vi "Trampsimple.vi"(6 "stop":bool, 7 "Rate [K/min]":dbl=0.05, 8 "delta K":dbl=0.2, 9 "T stop [K]":dbl=10.0 min=0.25 max=400.0, 10 "T start [K]":dbl=4.0 min=0.25 max=400.0, 11 "ITCSignal":T1={"ITC"=0, "Signal"=enum."Sensor 3"}) -> (2 "Finished":bool, 3 "ITCSignal out":T1={"ITC"=0, "Signal"=enum."Sensor 1"})   [LabVIEW 2011]
uses:
  Kelvinox drivers/ITCAPPS - Copie.LLB/ITCSignal.ctl
  Kelvinox drivers/ITCAPPS.LLB/ITCSignals.ctl
panel:
  out "Current T":dbl
  out "sign":i32=4 min=2 max=400
  out "timer":u32
  # "Sweep T"
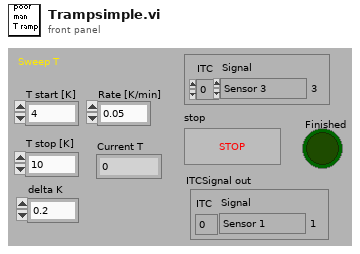
[diagram p1: front panel]
types:
  T1 = typedef "ITCSignal.ctl" = cluster{"ITC":u16, "Signal":T2}
  T2 = typedef "ITCSignals.ctl" = enum16{"Setpoint", "Sensor 1", "Sensor 2", "Sensor 3", "Needle Valve %", "Heater %"}
  T3 = typedef "ITCSetup.ctl" = cluster{"Description":string, "IO Info":T4}
  T4 = typedef "ITCIO.ctl" = cluster{"Address":T5, "Version":T6, "Ch 1 dec places":i16, "Ch 2 dec places":i16, "Ch 3 dec places":i16, "Ch1 Name":string, "Ch2 Name":string, "Ch3 Name":string}
  T5 = typedef "OxfordAddress.ctl" = cluster{"Com Port":i32, "ISOBUS Address":i32, "GPIB Address":i16, "Communication":enum16{"RS232", "ISOBUS", "GPIB", "Gateway"}}
  T6 = typedef "ITCVersion.ctl" = enum16{"ITC502", "ITC503", "ITC601"}
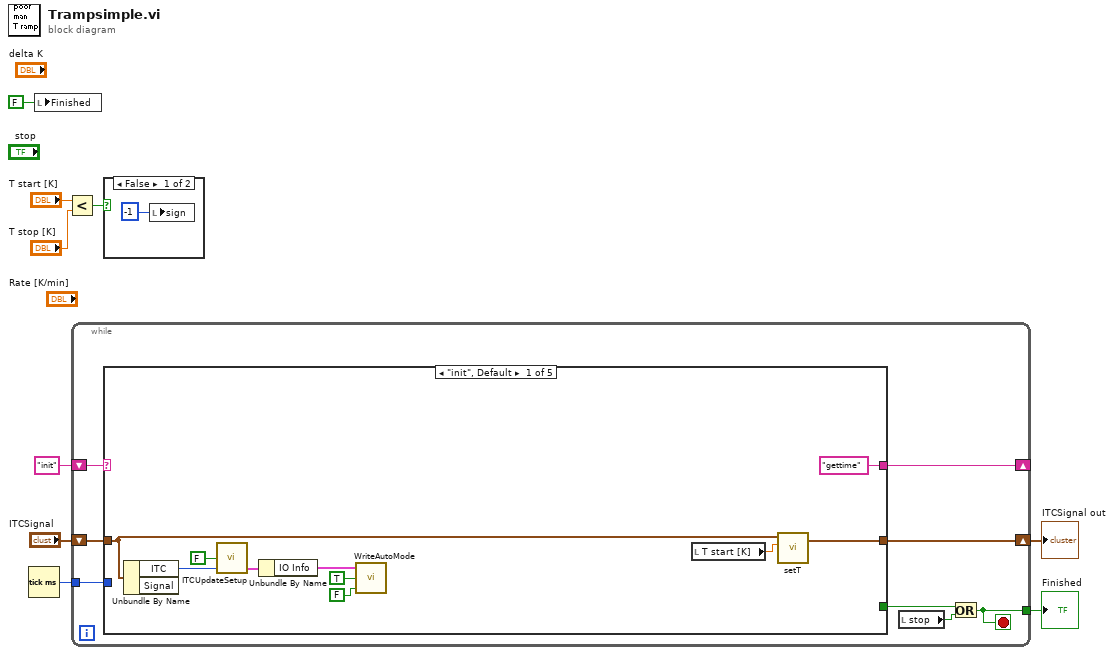
[diagram p0: block diagram]
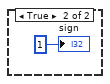
[diagram p2: hidden frame]
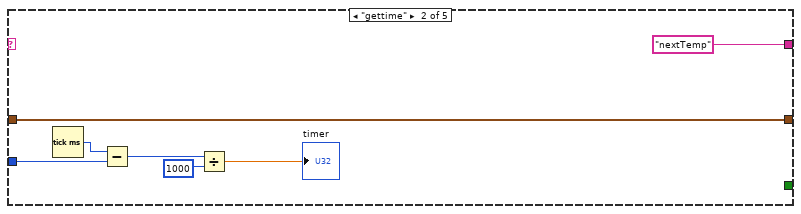
[diagram p3: hidden frame]
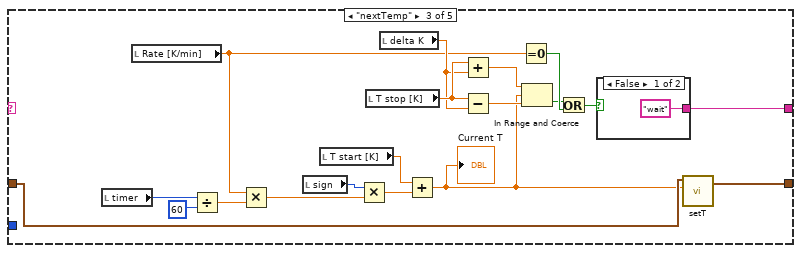
[diagram p4: hidden frame]
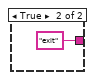
[diagram p5: hidden frame]
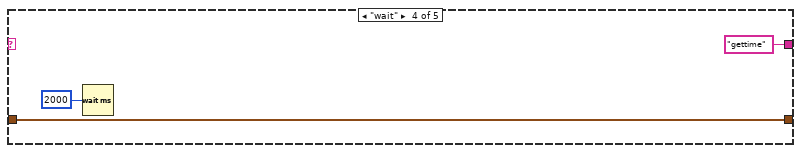
[diagram p6: hidden frame]
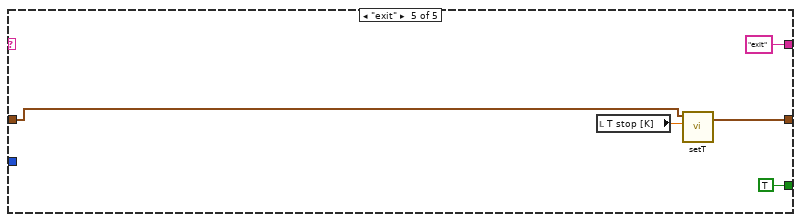
[diagram p7: hidden frame]
diagram:
  n1 = Tick Count (ms)() -> (millisecond timer value=w8:u32)
  n2 = local write "Finished"(FALSE ("Finished")) -> ()
  n3 = Less?(x="T start [K]", y="T stop [K]") -> (x < y?=w4:bool)
  n4 = while {
    shift-right: [w13] -> _
    shift-left: "init" -> [w17]
    tunnel: w8 -> [w16]
    shift-right: [w14] -> w2
    shift-left: "ITCSignal" -> [w15]
    tunnel: [w11] -> w3
    stop <- w11 stop-if-true
    n5 = case shown="\"init\", Default" w17 {
      tunnel: w16 -> [_ w33 _ _ _]
      tunnel: w15 -> [w21 w28 w49 w56 w60]
      tunnel: [w26 w28 w48 w56 w59] -> w14
      tunnel: [_ _ _ _ TRUE] -> w12
      tunnel: ["gettime" "nextTemp" w43 "gettime" "exit"] -> w13
      frame "init", Default {
        n6 = Unbundle By Name(w21) -> ("ITC"=w23:u16)  [unwired: 1 out]
        n7 = call "ITCUpdateSetup.vi"("Index"=w23, "Write to disk?"=FALSE) -> ("ITC Setup"=w22:T3)  [unwired: 2 in, 1 out]
        n8 = Unbundle By Name(w22) -> ("IO Info"=w20:T4)
        n9 = call "WriteAutoMode.vi"("Auto Needle Valve"=FALSE, "Auto Heat"=TRUE, "ITC IO Info"=w20) -> ()  [unwired: 1 out]
        n10 = local read "T start [K]"() -> (w27:dbl)
        n11 = call "setT.vi"("ITCSignal"=w21, "T target [K]"=w27) -> ("ITCSignal 2"=w26:T1)  [unwired: 3 in, 1 out]
      }
      frame "gettime" {
        n12 = Tick Count (ms)() -> (millisecond timer value=w34:u32)
        n13 = Subtract(x=w34, y=w33) -> (x-y=w32:u32)
        n14 = Divide(x=w32, y=u32 1000) -> (x/y=→"timer":dbl)
      }
      frame "nextTemp" {
        n15 = local read "timer"() -> (w41:u32)
        n16 = local read "Rate [K/min]"() -> (w38:dbl)
        n17 = Divide(x=w41, y=u32 60) -> (x/y=w39:dbl)
        n18 = Multiply(x=w38, y=w39) -> (x*y=w52:dbl)
        n19 = local read "sign"() -> (w51:i32)
        n20 = local read "T start [K]"() -> (w53:dbl)
        n21 = Multiply(x=w51, y=w52) -> (x*y=w50:dbl)
        n22 = local read "T stop [K]"() -> (w47:dbl)
        n23 = local read "delta K"() -> (w42:dbl)
        n24 = Add(x=w53, y=w50) -> (x+y=w44:dbl)
        "Current T" <- w44
        n25 = Add(x=w47, y=w42) -> (x+y=w46:dbl)
        n26 = Subtract(x=w47, y=w42) -> (x-y=w45:dbl)
        n27 = Equal To 0?(x=w38) -> (x = 0?=w37:bool)
        n28 = In Range and Coerce(upper limit=w46, x=w44, lower limit=w45) -> (In Range?=w36:bool)  [unwired: 1 out]
        n29 = Or(x=w36, y=w37) -> (x .or. y?=w35:bool)
        n30 = case shown="False" w35 {
          tunnel: ["wait" "exit"] -> w43
          frame False {
          }
          frame True {
          }
        }
        n31 = call "setT.vi"("ITCSignal"=w49, "T target [K]"=w44) -> ("ITCSignal 2"=w48:T1)  [unwired: 3 in, 1 out]
      }
      frame "wait" {
        n32 = Wait (ms)(milliseconds to wait=u32 2000) -> ()  [unwired: 1 out]
      }
      frame "exit" {
        n33 = local read "T stop [K]"() -> (w61:dbl)
        n34 = call "setT.vi"("ITCSignal"=w60, "T target [K]"=w61) -> ("ITCSignal 2"=w59:T1)  [unwired: 3 in, 1 out]
      }
    }
    n35 = local read "stop"() -> (w10:bool)
    n36 = Or(x=w12, y=w10) -> (x .or. y?=w11:bool)
  }
  "Finished" <- w3
  "ITCSignal out" <- w2
  n37 = case shown="False" w4 {
    frame False {
      n38 = local write "sign"(-1 ("sign")) -> ()
    }
    frame True {
      "sign" <- 1 ("sign")
    }
  }
